vi "Main Page.vi"(8 "error in (no error)":errorcluster, 11 "Node Ptr":T1 format="%.0x") -> (0 "error out":errorcluster)   [LabVIEW 2017, in "DSF System Explorer.lvlib"]
uses:
  DSF System Explorer.lvlib
  <vilib>/NI Veristand/Custom Device API/Custom Device Item Ref.ctl
  <vilib>/NI Veristand/Custom Device API/Custom Device API.lvlib
  Shared/DSF Shared.lvlib
panel:
  in  "Enable Thread Debugging":bool
  in  "Infinite FIFO Timeouts":bool
  in  "Measure Rx/Tx Durations":bool
  in  "Measure Period":bool
  in  "Refresh Configuration":bool
  in  "View Configuration":bool
  in  "DSF Configuration Path":path
  in  "Header":cluster{"Section Name":string}={"Section Name"="Data Sharing Framework Settings"}
  # "Debug Options"
  # "All Targets"
  # "Windows Only"
  # "Measurement Options"
  # "All Targets"
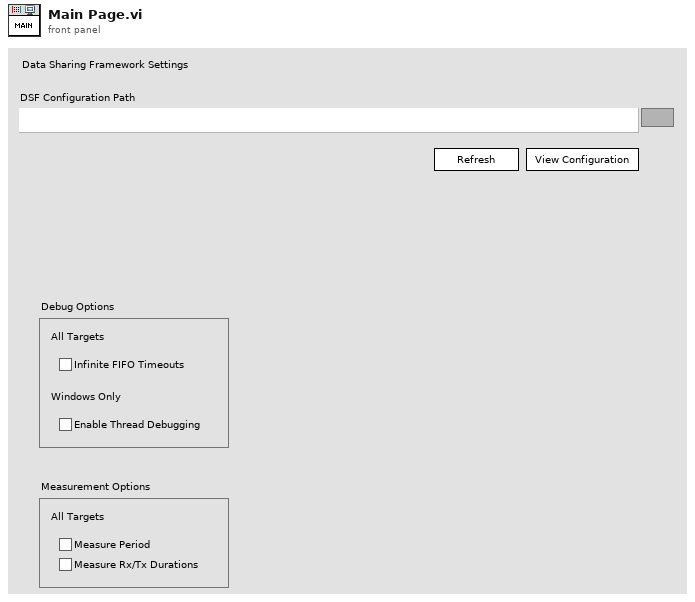
[diagram p1: front panel]
types:
  T1 = typedef "Custom Device API.lvlib/Custom Device Item Ref.ctl" = u64
  T2 = typedef "DSF Core.lvlibp/Framework.lvclass/Framework Options.ctl" = cluster{"FIFO Options":T3, "Thread Options":T4, "Plugin Options":T5, "Performance Options":T6}
  T3 = typedef "DSF Core.lvlibp/Framework.lvclass/DSF FIFO Options.ctl" = cluster{"Infinite Timeouts":bool}
  T4 = typedef "DSF Core.lvlibp/Thread.lvclass/Thread Options.ctl" = cluster{"Show FP On Call":bool, "Close FP After Call":bool, "Allow Debugging":bool, "Restart On Error":bool}
  T5 = typedef "DSF Core.lvlibp/Framework.lvclass/DSF Plugin Options.ctl" = cluster{"Default Components":bool}
  T6 = typedef "DSF Core.lvlibp/DSF Performance Options.ctl" = cluster{"Measure Period":bool, "Measure Rx/Tx Duration":bool}
  T7 = typedef "Custom Device API.lvlib/Custom Device Commands.ctl" = enum16{"Default", "Item renamed", "Shutdown", "Dynamic button pressed"}
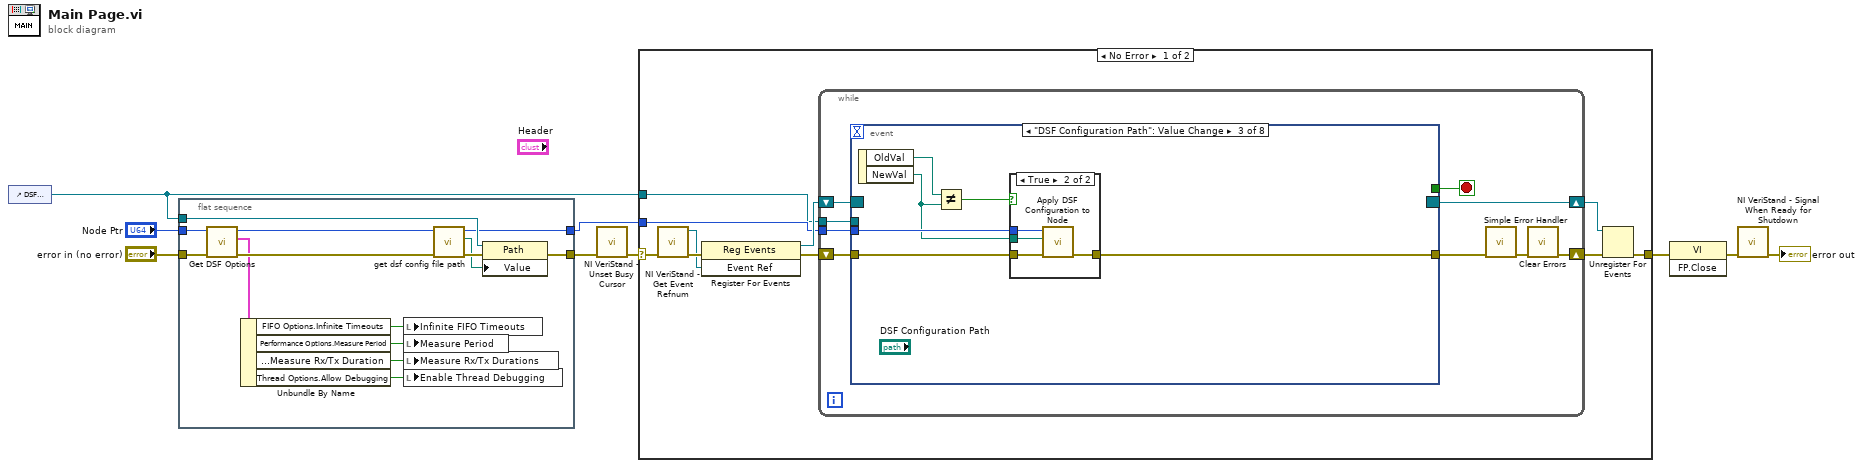
[diagram p0: block diagram]
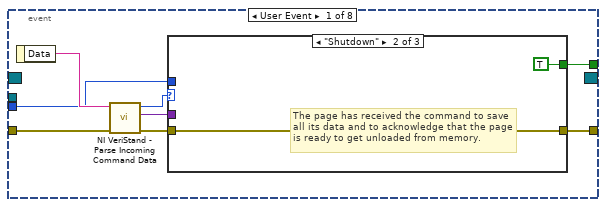
[diagram p2: hidden frame]
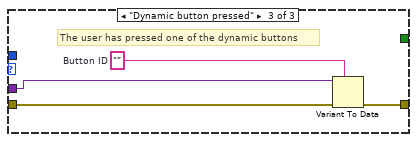
[diagram p4: hidden frame]
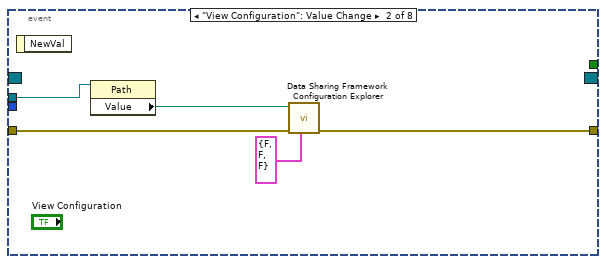
[diagram p5: hidden frame]
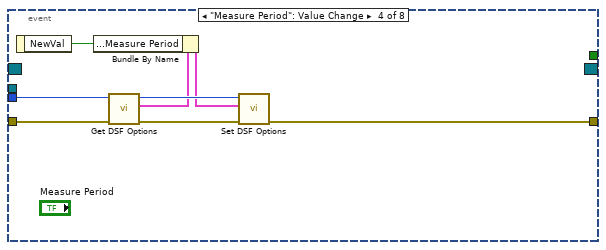
[diagram p7: hidden frame]
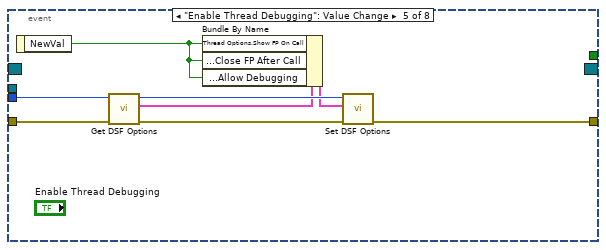
[diagram p8: hidden frame]
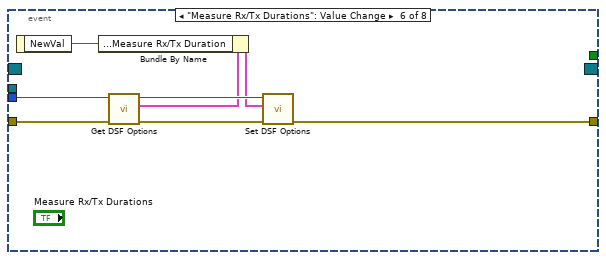
[diagram p9: hidden frame]
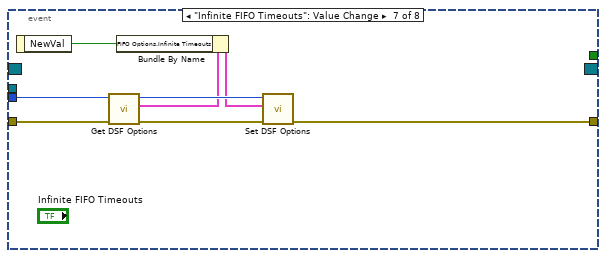
[diagram p10: hidden frame]
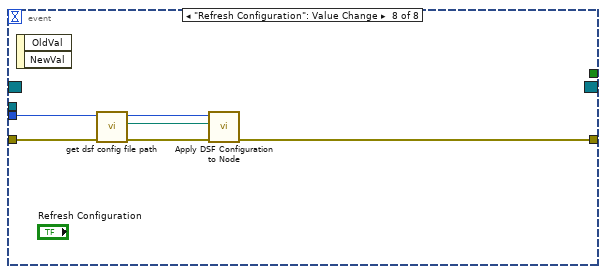
[diagram p11: hidden frame]
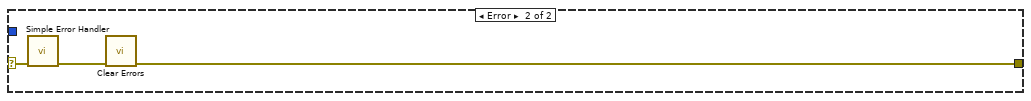
[diagram p12: hidden frame]
diagram:
  n1 = control-ref of="DSF Configuration Path"() -> (w1:refnum<vi>)
  n2 = flat-sequence "Initialization code" {
    tunnel: "error in (no error)" -> [w17]
    tunnel: "Node Ptr" -> [w18]
    tunnel: [w22] -> w5
    tunnel: [w20] -> w2
    tunnel: w1 -> [w21]
    frame #0 {
      n3 = call "Get DSF Options.vi"("error in (no error)"=w17, "Item Ref in"=w18) -> ("error out"=w15:errorcluster, "options"=w14:T2, "Item Ref out"=w16:T1)  [unwired: 7 in]
      n4 = Unbundle By Name(w14) -> ("FIFO Options.Infinite Timeouts"=w13:bool, "Performance Options.Measure Period"=w12:bool, "Performance Options.Measure Rx/Tx Duration"=w11:bool, "Thread Options.Allow Debugging"=w10:bool)
      n5 = local write "Infinite FIFO Timeouts"(w13) -> ()
      n6 = local write "Measure Period"(w12) -> ()
      n7 = local write "Measure Rx/Tx Durations"(w11) -> ()
      n8 = local write "Enable Thread Debugging"(w10) -> ()
      n9 = call "get dsf config file path.vi"("error in (no error)"=w15, "Node Ptr"=w16) -> ("error out"=w23:errorcluster, "Path"=w19:path, "Item Ref out"=w20:T1)  [unwired: 7 in]
      n10 = property class="Path"(reference=w21, error in=w23, "Value"=w19) -> (error out=w22:errorcluster)  [unwired: 1 out]
    }
  }
  n11 = call <vilib>:"NI VeriStand - Unset Busy Cursor.vi"("error in (no error)"=w5) -> ("error out"=w4:errorcluster)  [unwired: 10 out]
  n12 = case shown="No Error" w4 {
    selector: w4 -> [w25 w114]
    tunnel: [w30 w112] -> w9
    tunnel: w2 -> [w26 _]
    tunnel: w1 -> [w24 _]
    frame No Error {
      n13 = call <vilib>:"NI VeriStand - Get Event Refnum.vi"("error in (no error)"=w25) -> ("error out"=w33:errorcluster, "Event Ref"=w29:refnum<user-event>)  [unwired: 9 out]
      n14 = register-events(error in=w33, w29) -> (reference out=w27:refnum<event-registration>, error out=w28:errorcluster)  [unwired: 1 in]
      n15 = while {
        tunnel: w26 -> [w38]
        shift-right: [w35] -> w31
        shift-left: w28 -> [w41]
        shift-right: [w42] -> w32
        shift-left: w27 -> [w40]
        tunnel: w24 -> [w34]
        stop <- w39 stop-if-true
        n16 = event shown="[2] \"DSF Configuration Path\": Value Change" {
          selector: w40 -> [_ _ _ _ _ _ _ _]
          dyn-events: [_ _ _ _ _ _ _ _] -> w42
          timeout: _ -> [_ _ _ _ _ _ _ _]
          tunnel: w41 -> [w50 w62 w68 w79 w88 w95 w103 w111]
          tunnel: [w46 _ _ _ _ _ _ _] -> w39
          tunnel: [w45 w61 w66 w76 w85 w92 w100 w106] -> w37
          tunnel: w38 -> [w44 _ w67 w81 w89 w97 w105 w109]
          tunnel: w34 -> [_ w60 _ _ _ _ _ _]
          event User Event {
            n17 = event-data() -> ("Data"=w49:string)  [unwired: 1 out]
            n18 = call <vilib>:"NI VeriStand - Parse Incoming Command Data.vi"("error in (no error)"=w50, "Incoming data"=w49) -> ("error out"=w48:errorcluster, "Outgoing data"=w43:variant, "Action"=w47:T7)  [unwired: 7 out]
            n19 = case shown="\"Shutdown\"" w47 {
              tunnel: w48 -> [w51 w52 w57]
              tunnel: [_ TRUE _] -> w46
              tunnel: [w51 w52 w54] -> w45
              tunnel: w44 -> [_ _ _]
              tunnel: w43 -> [_ _ w56]
              frame "Default", Default {
              }
              frame "Shutdown" {
                # "The page has received the command to save all its data and to acknowledge that the page is ready to get unloaded from memory."
              }
              frame "Dynamic button pressed" {
                w55 = ""  # Button ID
                # "The user has pressed one of the dynamic buttons"
                n20 = Variant To Data(error in=w57, type=w55, Variant=w56) -> (error out=w54:errorcluster)  [unwired: 1 out]
              }
            }
          }
          event "View Configuration": Value Change {
            n21 = event-data() -> ()  [unwired: 2 out]
            n22 = property class="Path"(reference=w60) -> ("Value"=w59:path)  [unwired: 1 in, 2 out]
            n23 = call "Data Sharing Framework Configuration Explorer.vi"("menu options"=cluster{"open":bool, "save":bool, "view":bool} {"open"=FALSE, "save"=FALSE, "view"=FALSE}, "error in (no error)"=w62, "Path in"=w59) -> ("error out"=w61:errorcluster)  [unwired: 7 in, 1 out]
          }
          event "DSF Configuration Path": Value Change {
            n24 = event-data() -> ("OldVal"=w65:path, "NewVal"=w64:path)  [unwired: 1 out]
            n25 = Not Equal?(x=w65, y=w64) -> (x != y?=w63:bool)
            n26 = case shown="True" w63 {
              tunnel: w68 -> [w69 w73]
              tunnel: w67 -> [_ w70]
              tunnel: [w69 w72] -> w66
              tunnel: w64 -> [_ w71]
              frame False {
              }
              frame True {
                n27 = call "Apply DSF Configuration to Node.vi"("error in (no error)"=w73, "NewVal"=w71, "Item Ref in"=w70) -> ("error out"=w72:errorcluster)  [unwired: 8 in]
              }
            }
          }
          event "Measure Period": Value Change {
            n28 = event-data() -> ("NewVal"=w80:bool)  [unwired: 1 out]
            n29 = call "Get DSF Options.vi"("error in (no error)"=w79, "Item Ref in"=w81) -> ("error out"=w77:errorcluster, "options"=w74:T2, "Item Ref out"=w78:T1)  [unwired: 7 in]
            n30 = Bundle By Name(cluster=w74, "Performance Options.Measure Period"=w80) -> (w75:T2)
            n31 = call "Set DSF Options.vi"("error in (no error)"=w77, "options"=w75, "Item Ref in"=w78) -> ("error out"=w76:errorcluster)  [unwired: 7 in, 1 out]
          }
          event "Enable Thread Debugging": Value Change {
            n32 = event-data() -> ("NewVal"=w82:bool)  [unwired: 1 out]
            n33 = call "Get DSF Options.vi"("error in (no error)"=w88, "Item Ref in"=w89) -> ("error out"=w86:errorcluster, "options"=w83:T2, "Item Ref out"=w87:T1)  [unwired: 7 in]
            n34 = Bundle By Name(cluster=w83, "Thread Options.Show FP On Call"=w82, "Thread Options.Close FP After Call"=w82, "Thread Options.Allow Debugging"=w82) -> (w84:T2)
            n35 = call "Set DSF Options.vi"("error in (no error)"=w86, "options"=w84, "Item Ref in"=w87) -> ("error out"=w85:errorcluster)  [unwired: 7 in, 1 out]
          }
          event "Measure Rx/Tx Durations": Value Change {
            n36 = event-data() -> ("NewVal"=w96:bool)  [unwired: 1 out]
            n37 = call "Get DSF Options.vi"("error in (no error)"=w95, "Item Ref in"=w97) -> ("error out"=w93:errorcluster, "options"=w90:T2, "Item Ref out"=w94:T1)  [unwired: 7 in]
            n38 = Bundle By Name(cluster=w90, "Performance Options.Measure Rx/Tx Duration"=w96) -> (w91:T2)
            n39 = call "Set DSF Options.vi"("error in (no error)"=w93, "options"=w91, "Item Ref in"=w94) -> ("error out"=w92:errorcluster)  [unwired: 7 in, 1 out]
          }
          event "Infinite FIFO Timeouts": Value Change {
            n40 = event-data() -> ("NewVal"=w104:bool)  [unwired: 1 out]
            n41 = call "Get DSF Options.vi"("error in (no error)"=w103, "Item Ref in"=w105) -> ("error out"=w101:errorcluster, "options"=w98:T2, "Item Ref out"=w102:T1)  [unwired: 7 in]
            n42 = Bundle By Name(cluster=w98, "FIFO Options.Infinite Timeouts"=w104) -> (w99:T2)
            n43 = call "Set DSF Options.vi"("error in (no error)"=w101, "options"=w99, "Item Ref in"=w102) -> ("error out"=w100:errorcluster)  [unwired: 7 in, 1 out]
          }
          event "Refresh Configuration": Value Change {
            n44 = event-data() -> ()  [unwired: 3 out]
            n45 = call "get dsf config file path.vi"("error in (no error)"=w111, "Node Ptr"=w109) -> ("error out"=w110:errorcluster, "Path"=w107:path, "Item Ref out"=w108:T1)  [unwired: 7 in]
            n46 = call "Apply DSF Configuration to Node.vi"("error in (no error)"=w110, "NewVal"=w107, "Item Ref in"=w108) -> ("error out"=w106:errorcluster)  [unwired: 8 in]
          }
        }
        n47 = call <vilib>:"Simple Error Handler.vi"("error in (no error)"=w37) -> ("error out"=w36:errorcluster)  [unwired: 1 in, 7 out]
        n48 = call <vilib>:"Clear Errors.vi"("error in (no error)"=w36) -> ("error out"=w35:errorcluster)  [unwired: 1 in, 5 out]
      }
      n49 = Unregister For Events(event registration refnum=w32, error in=w31) -> (error out=w30:errorcluster)
    }
    frame Error {
      n50 = call <vilib>:"Simple Error Handler.vi"("error in (no error)"=w114) -> ("error out"=w113:errorcluster)  [unwired: 1 in, 7 out]
      n51 = call <vilib>:"Clear Errors.vi"("error in (no error)"=w113) -> ("error out"=w112:errorcluster)  [unwired: 1 in, 5 out]
    }
  }
  n52 = invoke class="VI" method="FP.Close"(error in=w9) -> (error out=w8:errorcluster)  [unwired: 2 in, 2 out]
  n53 = call <vilib>:"NI VeriStand - Signal When Ready for Shutdown.vi"("error in (no error)"=w8) -> ("error out"=→"error out":errorcluster)  [unwired: 10 out]
